vi "Quit.vi"(8 "No Error":errorcluster) -> (0 "error out":errorcluster)   [LabVIEW 2026, in "SDL3.lvlib" / "Init.lvlib"]
doc: "<B>Summary</B>\nClean up all initialized subsystems.\n\n<B>Remarks</B>\nYou should call this function even if you have already shutdown each initialized subsystem with <B>SDL_QuitSubSystem()</B>. It is safe to call this function even in the case of errors in initialization.\n\nYou can use this function with <B>atexit()</B> to ensure that it is run when your application is shutdown, but it is not wise to do this from a library or other dynamically loaded code."
uses:
  Init.lvlib
  Lib/SDL3.dll
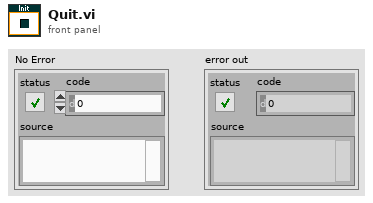
[diagram p1: front panel]
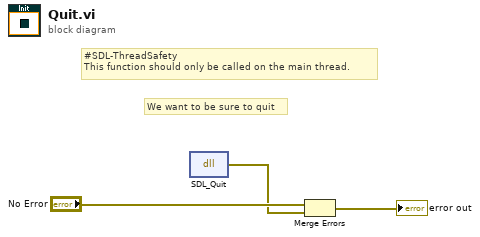
[diagram p0: block diagram]
diagram:
  # "#SDL-ThreadSafety\nThis function should only be called on the main thread."
  # "We want to be sure to quit"
  n1 = dll-call lib="C:/Users/saukko/Dev/LV-SDL3/Sources/SDL3/Lib/SDL3.*" fn="SDL_Quit"() -> (error out=w1:errorcluster)  [unwired: 4 in, 1 out]
  n2 = Merge Errors("No Error", w1) -> (→"error out":errorcluster)
